vi "myRIO_BRig_RT__Case_Exp_State_Selection__v5.vi"(0 "input_dataCurrent":u16[](array[numeric]), 1 "input_state":T1, 2 "input_dataExp":u16[](array[numeric]), 5 "input_LickL":bool, 7 "input_FPGA_SelectReward":bool, 9 "input_FPGA_SelectWrong":bool, 11 "input_LickR":bool, 12 "input_arrTrig":bool[](array[boolean])) -> (3 "output_state":T1, 4 "output_dataCurrent":u16[](array[numeric]), 10 "output_LC_Event_l1":bool, 13 "output_LC_Laser_l2":bool, 14 "output_LC_Event_l2":bool, 15 "output_LC_Laser_l1":bool)   [LabVIEW 2014]
uses:
  myRIO_BRig_RT__Case_Exp_stateList.ctl
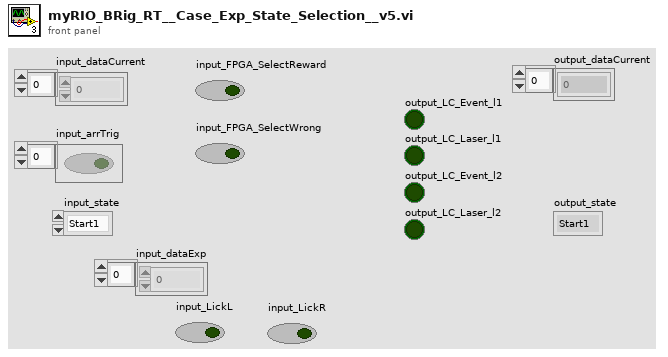
[diagram p1: front panel]
types:
  T1 = typedef "myRIO_BRig_RT__Case_Exp_stateList.ctl" = enum16{"Start1", "Start2", "Start3", "saveSettings1", "saveSettings2", "saveSettings3", "saveSettings4", "saveSettings_LC_ENL_l1", "saveSettings_LC_ENL_l2", "saveSettings_LC_Cue_l1", "saveSettings_LC_Cue_l2", "saveSettings6_LC_l1_Other", "SaveSettings6_LC_l2_Other", "setSettings_Audio", "setSettings_Laser", "initBlock_pre", "initBlock", "initBlock2", "initBlock_post", "initTrial_pre", "initTrial", "initTrial2", "initTrial3", "initTrial4", "initTrial_LC_ENL1", "initTrial_LC_Cue1", "initTrial_LC_Cue1_2", "initTrial_LC_Sel", "initTrial_post", "ENL1_pre", "ENL1", "ENL1_post", "ENL1Penalty_pre", "ENL1Penalty", "ENL2_pre", "ENL2", "ENL2Penalty_pre", "ENL2Penalty", "Cue1_pre", "Cue1", "Cue1_post", "Cue1Penalty_pre", "Cue1Penalty", "Cue2_pre", "Cue2", "Cue2Penalty_pre", "Cue2Penalty", "Selection_pre", "Selection", "Select_post", "SelectReward_pre", "SelectReward", "SelectRewardPost_pre", "SelectRewardPost", "SelectWrong_pre", "SelectWrong", "SelectWrong_post", "SelectTimeout_pre", "SelectTimeout", "SelectTimeout_post", "endTrial_pre", "endTrial1", "endTrial2", "endTrial3", "endTrial_post", "endBlock_pre", "endBlock", "endBlock_post", "endExp", "commConnect", "commUpload_pre", "commUpload_dataBlock", "commUpload_dataCurrent", "commUpload_dataExp", "commUpload_dataLC", "commUpload_dataTrial", "commUpload_post", "saveData_pre", "saveData_dataBlock", "saveData_dataCurrent", "saveData_dataExp", "saveData_dataLC", "saveData_dataTrial", "saveData_post", "empty_endBlock1", "empty_endBlock2", "empty_endTrial1", "empty_endTrial2", "empty_endTrial3", "empty_endTrial4", "empty_endTrial5", "dummyState", "dummyState_endBlock"}
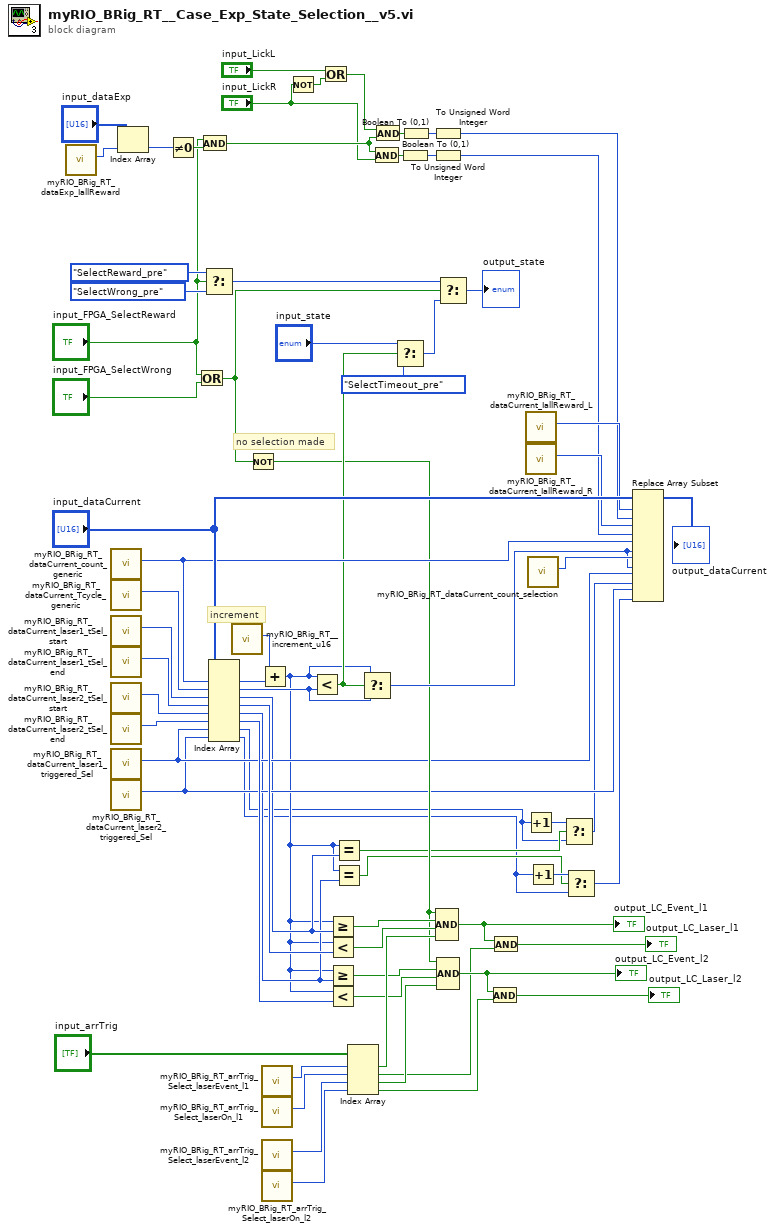
[diagram p0: block diagram]
diagram:
  # "no selection made"
  # "increment"
  n1 = call "myRIO_BRig_RT_dataExp_IallReward.vi"() -> ("output_I_allReward"=w15:i32)  [unwired: 11 in]
  n2 = call "myRIO_BRig_RT_dataCurrent_count_generic.vi"() -> ("output_count_generic"=w56:i32)  [unwired: 11 in]
  n3 = call "myRIO_BRig_RT_dataCurrent_Tcycle_generic.vi"() -> ("output_Tcycle_generic"=w68:i32)  [unwired: 11 in]
  n4 = call "myRIO_BRig_RT_dataCurrent_laser1_tSel_start.vi"() -> ("output_laser1_tSel_start"=w69:i32)  [unwired: 11 in]
  n5 = call "myRIO_BRig_RT_dataCurrent_laser1_tSel_end.vi"() -> ("output_laser1_tSel_end"=w70:i32)  [unwired: 11 in]
  n6 = call "myRIO_BRig_RT_dataCurrent_laser2_tSel_start.vi"() -> ("output_laser2_tSel_start"=w61:i32)  [unwired: 11 in]
  n7 = call "myRIO_BRig_RT_dataCurrent_laser2_tSel_end.vi"() -> ("output_laser2_tSel_end"=w60:i32)  [unwired: 11 in]
  n8 = call "myRIO_BRig_RT_dataCurrent_laser1_triggered_Sel.vi"() -> ("output_laser1_triggered_Selection"=w31:i32)  [unwired: 11 in]
  n9 = call "myRIO_BRig_RT_dataCurrent_laser2_triggered_Sel.vi"() -> ("output_laser2_triggered_Selection"=w30:i32)  [unwired: 11 in]
  n10 = Index Array(array="input_dataExp", index=w15) -> (element=w17:u16)
  n11 = Not Equal To 0?(x=w17) -> (x != 0?=w16:bool)
  n12 = Or(x="input_FPGA_SelectReward", y="input_FPGA_SelectWrong") -> (x .or. y?=w50:bool)
  n13 = And(x="input_FPGA_SelectReward", y=w16) -> (x .and. y?=w9:bool)
  n14 = Select(t=myRIO_BRig_RT__Case_Exp_stateList."SelectReward_pre" ("Enum"), s="input_FPGA_SelectReward", f=myRIO_BRig_RT__Case_Exp_stateList."SelectWrong_pre" ("Enum")) -> (s? t:f=w71:T1)
  n15 = Index Array(array="input_dataCurrent", index #1=w56, index #2=w68, index #3=w69, index #4=w70, index #5=w61, index #6=w60, index #7=w31, index #8=w30) -> (element #1=w66:u16, element #2=w54:u16, element #3=w29:u16, element #4=w59:u16, element #5=w28:u16, element #6=w58:u16, element #7=w24:u16, element #8=w21:u16)
  n16 = call "myRIO_BRig_RT__increment_u16.vi"() -> ("output_increment__u16"=w67:u16)  [unwired: 11 in]
  n17 = Not(x=w50) -> (.not. x?=w43:bool)
  n18 = Add(x=w67, y=w66) -> (x+y=w27:u16)
  n19 = call "myRIO_BRig_RT_arrTrig_Select_laserEvent_l1.vi"() -> ("output_arrTrig_Select_laserEvent_l1"=w46:i32)  [unwired: 11 in]
  n20 = call "myRIO_BRig_RT_arrTrig_Select_laserOn_l1.vi"() -> ("output_arrTrig_Select_laserOn_l1"=w45:i32)  [unwired: 11 in]
  n21 = call "myRIO_BRig_RT_arrTrig_Select_laserEvent_l2.vi"() -> ("output_arrTrig_Select_laserEvent_l2"=w33:i32)  [unwired: 11 in]
  n22 = call "myRIO_BRig_RT_arrTrig_Select_laserOn_l2.vi"() -> ("output_arrTrig_Select_laserOn_l2"=w32:i32)  [unwired: 11 in]
  n23 = Not(x="input_LickR") -> (.not. x?=w2:bool)
  n24 = Less?(x=w27, y=w54) -> (x < y?=w55:bool)
  n25 = Or(x="input_LickL", y=w2) -> (x .or. y?=w1:bool)
  n26 = Greater Or Equal?(x=w27, y=w29) -> (x >= y?=w49:bool)
  n27 = Less?(x=w27, y=w59) -> (x < y?=w48:bool)
  n28 = Greater Or Equal?(x=w27, y=w28) -> (x >= y?=w42:bool)
  n29 = Less?(x=w27, y=w58) -> (x < y?=w41:bool)
  n30 = Equal?(x=w27, y=w29) -> (x = y?=w26:bool)
  n31 = Equal?(x=w27, y=w28) -> (x = y?=w22:bool)
  n32 = Index Array(array="input_arrTrig", index #1=w46, index #2=w45, index #3=w33, index #4=w32) -> (element #1=w44:bool, element #2=w36:bool, element #3=w40:bool, element #4=w38:bool)
  n33 = Select(t=w27, s=w55, f=w54) -> (s? t:f=w52:u16)
  n34 = And(x=w9, y="input_LickR") -> (x .and. y?=w12:bool)
  n35 = And(x=w1, y=w9) -> (x .and. y?=w13:bool)
  n36 = Select(t="input_state", s=w55, f=myRIO_BRig_RT__Case_Exp_stateList."SelectTimeout_pre" ("Enum")) -> (s? t:f=w63:T1)
  n37 = Boolean To (0,1)(Boolean=w12) -> (0, 1=w10:i16)
  n38 = Boolean To (0,1)(Boolean=w13) -> (0, 1=w11:i16)
  n39 = To Unsigned Word Integer(number=w11) -> (unsigned 16bit integer=w6:u16)
  n40 = To Unsigned Word Integer(number=w10) -> (unsigned 16bit integer=w5:u16)
  n41 = Compound Arithmetic op=AND(w43, w49, w48, w44) -> (w37:bool)
  "output_LC_Event_l1" <- w37
  n42 = Compound Arithmetic op=AND(w43, w42, w41, w40) -> (w39:bool)
  "output_LC_Event_l2" <- w39
  n43 = Select(t=w71, s=w50, f=w63) -> (s? t:f=→"output_state":T1)
  n44 = And(x=w39, y=w38) -> (x .and. y?=→"output_LC_Laser_l2":bool)
  n45 = And(x=w37, y=w36) -> (x .and. y?=→"output_LC_Laser_l1":bool)
  n46 = call "myRIO_BRig_RT_dataCurrent_IallReward_L.vi"() -> ("output_IallReward_L"=w8:i32)  [unwired: 11 in]
  n47 = call "myRIO_BRig_RT_dataCurrent_IallReward_R.vi"() -> ("output_IallReward_R"=w7:i32)  [unwired: 11 in]
  n48 = Increment(x=w24) -> (x+1=w25:u16)
  n49 = call "myRIO_BRig_RT_dataCurrent_count_selection.vi"() -> ("output_count_generic"=w53:i32)  [unwired: 11 in]
  n50 = Increment(x=w21) -> (x+1=w23:u16)
  n51 = Select(t=w25, s=w26, f=w24) -> (s? t:f=w20:u16)
  n52 = Select(t=w23, s=w22, f=w21) -> (s? t:f=w19:u16)
  n53 = Replace Array Subset(array="input_dataCurrent", new element #1=w6, index #1=w8, new element #2=w5, index #2=w7, new element #3=w52, index #3=w56, new element #4=w52, index #4=w53, new element #5=w20, index #5=w31, new element #6=w19, index #6=w30) -> (→"output_dataCurrent":u16[])
